vi "Flywheel_Hardware_Begin.vi"(8 "error in":errorcluster) -> (0 "error out":errorcluster)   [LabVIEW 2020]
uses:
  <vilib>/Rock Robotics/WPI/ThirdParty/Phoenix-LabVIEW/Motor Controller/Controls/CTRE_Phoenix_MotorControl_SupplyCurrentLimitConfiguration.ctl
  <vilib>/Rock Robotics/WPI/ThirdParty/Phoenix-LabVIEW/Motor Controller/Controls/CTRE_Phoenix_MotorControl_NeutralMode.ctl
  <vilib>/Rock Robotics/WPI/ThirdParty/Phoenix-LabVIEW/Motor Controller/Controls/CTRE_Phoenix_MotorControl_TalonFXInvertType.ctl
  Flywheel_Hardware_Globals.vi
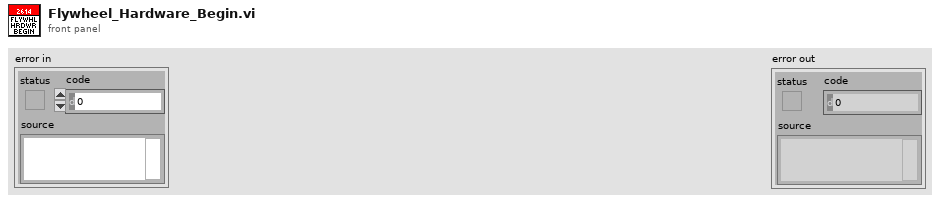
[diagram p1: front panel]
types:
  T1 = typedef "CTRE_Phoenix_MotorControl_TalonFXInvertType.ctl" = enum16{"Counter-Clockwise", "Clockwise"}
  T2 = typedef "CTRE_Phoenix_MotorControl_NeutralMode.ctl" = enum8{"EEPROMSetting", "Override to Coast", "Override to Brake"}
  T3 = typedef "CTRE_Phoenix_MotorControl_SupplyCurrentLimitConfiguration.ctl" = cluster{"Enable?":bool, "Current Limit":dbl, "Threshold Current":dbl, "Threshold Time":dbl}
  T4 = typedef "WPI_MotorControlDeviceRef.ctl" = cluster{"DeviceStatus":errorcluster, "Type":T5, "PWM":cluster{"PWM Channel":T6, "DeadBand":T7}, "CAN":cluster{"Device Number":u8, "SetOutput VI Ref":variant, "GetOutput VI Ref":variant, "Enable VI Ref":variant, "Disable VI Ref":variant, "Data":variant}, "Invert":bool, "DIO PWM":cluster{"PWM \"Enable\" Channel":T6, "DIOChannel":T8, "PWM Rate":dbl}}
  T5 = typedef "WPI_MotorControlType.ctl" = enum16{"PWM", "CAN", "DIO PWM"}
  T6 = typedef "FPGA_DIOPWMChannel.ctl" = enum8{"PWM 0", "PWM 1", "PWM 2", "PWM 3", "PWM 4", "PWM 5", "PWM 6", "PWM 7", "PWM 8", "PWM 9", "PWM MXP 0", "PWM MXP 1", "PWM MXP 2", "PWM MXP 3", "PWM MXP 4", "PWM MXP 5", "PWM MXP 6", "PWM MXP 7", "PWM MXP 8", "PWM MXP 9", "Invalid"}
  T7 = typedef "WPI_PWMDeadband.ctl" = cluster{"Name":string, "maxPositivePwm":i32, "minPositivePwm":i32, "centerPwm":i32, "maxNegativePwm":i32, "minNegativePwm":i32, "angularRange":u16}
  T8 = typedef "FPGA_DIOChannel.ctl" = enum8{"DIO 0", "DIO 1", "DIO 2", "DIO 3", "DIO 4", "DIO 5", "DIO 6", "DIO 7", "DIO 8", "DIO 9", "DIO MXP 0", "DIO MXP 1", "DIO MXP 2", "DIO MXP 3", "DIO MXP 4", "DIO MXP 5", "DIO MXP 6", "DIO MXP 7", "DIO MXP 8", "DIO MXP 9", "DIO MXP 10", "DIO MXP 11", "DIO MXP 12", "DIO MXP 13", "DIO MXP 14", "DIO MXP 15", "SPI Port CS1", "SPI Port CS2", "SPI Port CS3", "SPI Port MISO", "SPI Port MOSI", "Invalid"}
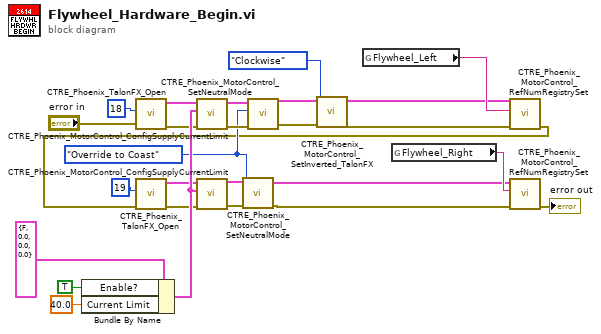
[diagram p0: block diagram]
diagram:
  w9 = CTRE_Phoenix_MotorControl_NeutralMode."Override to Coast" ("Motor Control Neutral Mode")
  n1 = Bundle By Name(cluster=T3 {"Enable?"=FALSE, "Current Limit"=0.0, "Threshold Current"=0.0, "Threshold Time"=0.0} ("Supply Current Limit Configuration"), "Enable?"=TRUE, "Current Limit"=40.0) -> (w22:T3)
  n2 = call <vilib>:"CTRE_Phoenix_TalonFX_Open.vi"("error in"="error in", "Device Number"=u8 18) -> ("error out"=w19:errorcluster, "PhoenixMotorControlDevRef"=w20:T4)  [unwired: 8 in]
  n3 = call <vilib>:"CTRE_Phoenix_MotorControl_ConfigSupplyCurrentLimit.vi"("error in (no error)"=w19, "Supply Current Limit Configuration"=w22, "PhoenixMotorControlDevRef"=w20) -> ("error out"=w10:errorcluster, "PhoenixMotorControlDevRef"=w11:T4)  [unwired: 7 in]
  n4 = call <vilib>:"CTRE_Phoenix_MotorControl_SetNeutralMode.vi"("error in (no error)"=w10, "Motor Control Neutral Mode"=w9, "PhoenixMotorControlDevRef"=w11) -> ("error out"=w8:errorcluster, "PhoenixMotorControlDevRef"=w7:T4)  [unwired: 7 in]
  n5 = call <vilib>:"CTRE_Phoenix_MotorControl_SetInverted_TalonFX.vi"("error in (no error)"=w8, "Invert Type"=CTRE_Phoenix_MotorControl_TalonFXInvertType."Clockwise", "PhoenixMotorControlDevRef"=w7) -> ("error out"=w4:errorcluster, "PhoenixMotorControlDevRef"=w5:T4)  [unwired: 7 in]
  n6 = global read "Flywheel_Hardware_Globals.vi" "Flywheel_Left"() -> (w17:string)
  n7 = global read "Flywheel_Hardware_Globals.vi" "Flywheel_Right"() -> (w16:string)
  n8 = call <vilib>:"CTRE_Phoenix_MotorControl_RefNumRegistrySet.vi"("error in (no error)"=w4, "refnum name"=w17, "PhoenixMotorControlDevRef"=w5) -> ("error out"=w3:errorcluster)  [unwired: 7 in, 1 out]
  n9 = call <vilib>:"CTRE_Phoenix_TalonFX_Open.vi"("error in"=w3, "Device Number"=u8 19) -> ("error out"=w18:errorcluster, "PhoenixMotorControlDevRef"=w21:T4)  [unwired: 8 in]
  n10 = call <vilib>:"CTRE_Phoenix_MotorControl_ConfigSupplyCurrentLimit.vi"("error in (no error)"=w18, "Supply Current Limit Configuration"=w22, "PhoenixMotorControlDevRef"=w21) -> ("error out"=w14:errorcluster, "PhoenixMotorControlDevRef"=w15:T4)  [unwired: 7 in]
  n11 = call <vilib>:"CTRE_Phoenix_MotorControl_SetNeutralMode.vi"("error in (no error)"=w14, "Motor Control Neutral Mode"=w9, "PhoenixMotorControlDevRef"=w15) -> ("error out"=w13:errorcluster, "PhoenixMotorControlDevRef"=w12:T4)  [unwired: 7 in]
  n12 = call <vilib>:"CTRE_Phoenix_MotorControl_RefNumRegistrySet.vi"("error in (no error)"=w13, "refnum name"=w16, "PhoenixMotorControlDevRef"=w12) -> ("error out"=→"error out":errorcluster)  [unwired: 7 in, 1 out]
